vi "Enable Zero Correct.vi"(8 "error in (no error)":errorcluster, 10 "Enable Zero Correct (F: Disable)":bool, 11 "VISA resource name":refnum<visa-resource-name>) -> (0 "error out":errorcluster, 3 "VISA resource name out":refnum<visa-resource-name>)   [LabVIEW 2019, in "Keithley 6517.lvlib"]
doc: "Enables or Disables Zero Correct.\n\nZero correct algebraically subtracts the voltage offset term from the measurement."
uses:
  Keithley 6517.lvlib
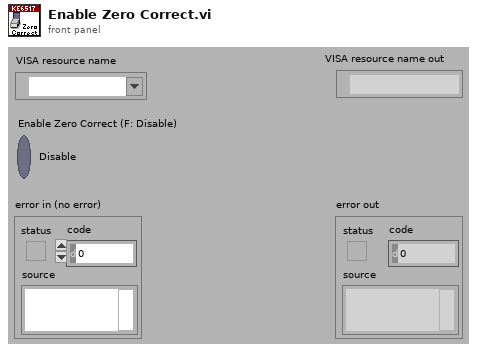
[diagram p1: front panel]
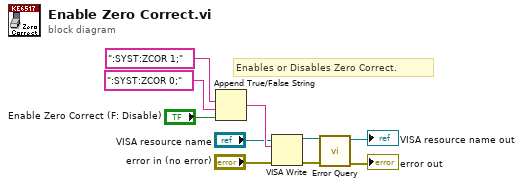
[diagram p0: block diagram]
diagram:
  # "Enables or Disables Zero Correct."
  n1 = Append True/False String(1:"Enable Zero Correct (F: Disable)", 2:":SYST:ZCOR 0;" ("command"), 3:":SYST:ZCOR 1;" ("command")) -> (0:w7:string)  [unwired: 1 in]
  n2 = VISA Write(VISA resource name="VISA resource name", write buffer=w7, error in (no error)="error in (no error)") -> (VISA resource name out=w5:refnum<visa-resource-name>, error out=w6:errorcluster)  [unwired: 1 out]
  n3 = call "Error Query.vi"("error in (no error)"=w6, "VISA resource name"=w5) -> ("error out"=→"error out":errorcluster, "VISA resource name out"=→"VISA resource name out":refnum<visa-resource-name>)  [unwired: 6 in, 2 out]
